vi "niRFUtil TRC Save Traces to File (Single Trace, 1D).vi"(0 "File Path In (dialog if empty)":T2, 1 "Append to File? (new file:F)":bool, 5 "Measurement Trace":T1 format="%.2f", 7 "Forma (%.12f)":T4="%.12f", 9 "Delimiter (\\t)":T3="\t", 11 "error in":errorcluster, 12 "Transpose? (no:F)":bool) -> (15 "error out":errorcluster)   [LabVIEW 2015, in "niRFUtil.lvlib"]
uses:
  niRFUtil.lvlib
  Includes/niRFUtil INC File Path.ctl
  Includes/niRFUtil INC Text File Format Specifier.ctl
  Includes/niRFUtil INC Text File Delimiter.ctl
  Includes/niRFUtil INC Trace.ctl
panel:
  out "File Path Out":T2
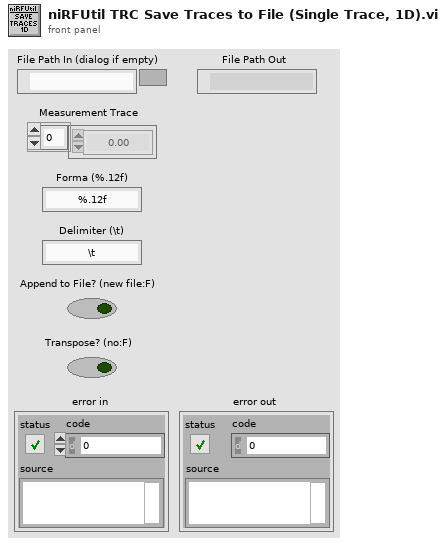
[diagram p1: front panel]
types:
  T1 = typedef "niRFUtil.lvlib/niRFUtil INC Trace.ctl" = sgl[]
  T2 = typedef "niRFUtil.lvlib/niRFUtil INC File Path.ctl" = path
  T3 = typedef "niRFUtil.lvlib/niRFUtil INC Text File Delimiter.ctl" = string
  T4 = typedef "niRFUtil.lvlib/niRFUtil INC Text File Format Specifier.ctl" = string
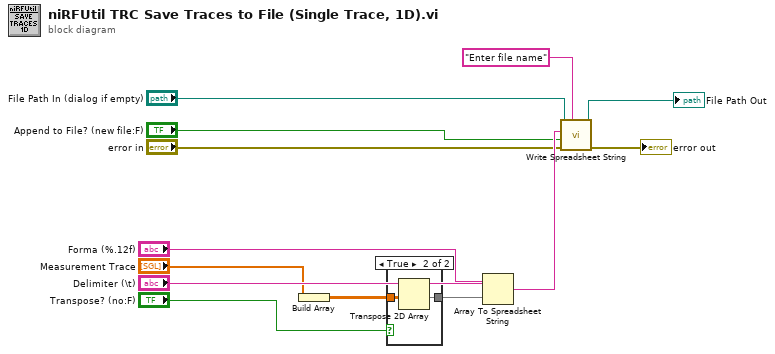
[diagram p0: block diagram]
diagram:
  n1 = Build Array("Measurement Trace") -> (w3:sgl[][])
  n2 = case shown="True" "Transpose? (no:F)" {
    tunnel: [w14 w16] -> w13
    tunnel: w3 -> [w14 w15]
    frame False {
    }
    frame True {
      n3 = Transpose 2D Array(2D array=w15) -> (transposed array=w16:sgl[][])
    }
  }
  n4 = Array To Spreadsheet String(delimiter (Tab)="Delimiter (\\t)", array=w13, 3:"Forma (%.12f)") -> (spreadsheet string=w11:string)
  n5 = call <vilib>:"Write Spreadsheet String.vi"("prompt"="Enter file name", "error in"="error in", "append to file? (new file:F)"="Append to File? (new file:F)", "spreadsheet string"=w11, "file path (dialog if empty)"="File Path In (dialog if empty)") -> ("error out"=→"error out":errorcluster, "path"=→"File Path Out":path)  [unwired: 2 in, 3 out]
